vi "AskForExperimentPostNotes.vi"(7 "String Control":string) -> (0 "Disable Button 2":bool, 1 "Experiment Name 2":string)   [LabVIEW 2024]
panel:
  in  "Disable Button":bool
  in  "OK Button":bool
  in  "Post Experiment Notes":string
  # "Please provide notes on the result of the experiment."
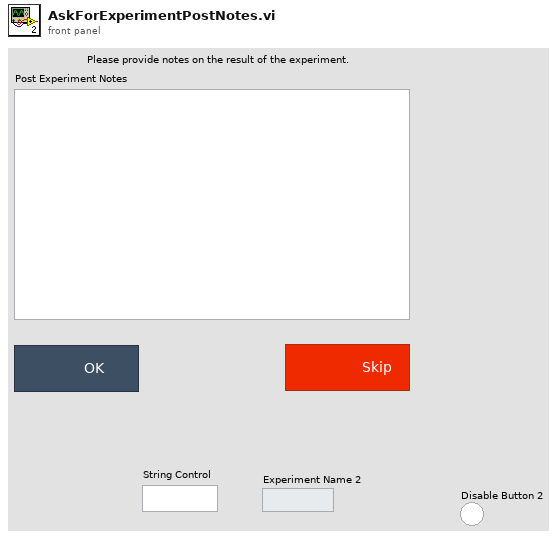
[diagram p1: front panel]
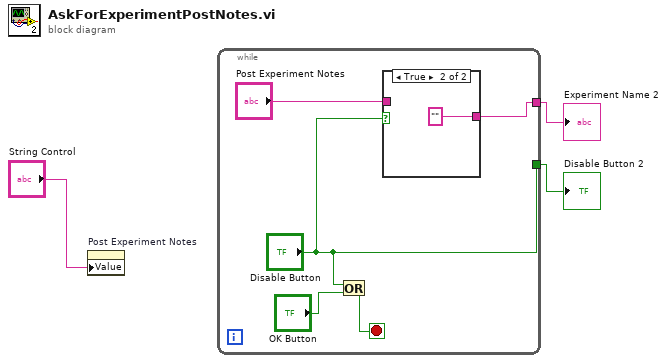
[diagram p0: block diagram]
diagram:
  n1 = property on="Post Experiment Notes" class="Str"("Value"="String Control") -> ()  [unwired: 2 in, 2 out]
  n2 = while {
    tunnel: [w5] -> w2
    tunnel: ["Disable Button"] -> w1
    stop <- w7 stop-if-true
    n3 = Or(x="Disable Button", y="OK Button") -> (x .or. y?=w7:bool)
    n4 = case shown="True" "Disable Button" {
      tunnel: [w9 "" ("Experiment Description")] -> w5
      tunnel: "Post Experiment Notes" -> [w9 _]
      frame False {
      }
      frame True {
      }
    }
  }
  "Experiment Name 2" <- w2
  "Disable Button 2" <- w1
